vi "Node - Writer.vi"(8 "error in (no error)":errorcluster, 11 "Node Data In":T1) -> (0 "error out":errorcluster, 3 "Node Data Out":T1)   [LabVIEW 2016, in "PXImc Router.lvlib"]
uses:
  PXImc Router.lvlib
  Controls/Node Data.ctl
  Controls/Node/Node - PXImc Parameters.ctl
  Controls/Node/Node - Writer Data.ctl
  Controls/Node/Node Ch Properties.ctl
  Controls/Data Type.ctl
  Controls/Node/Node - Readers Data.ctl
  Controls/Node/Node - Reader Data.ctl
  Engine/PXImc Custom Device Engine.lvlib
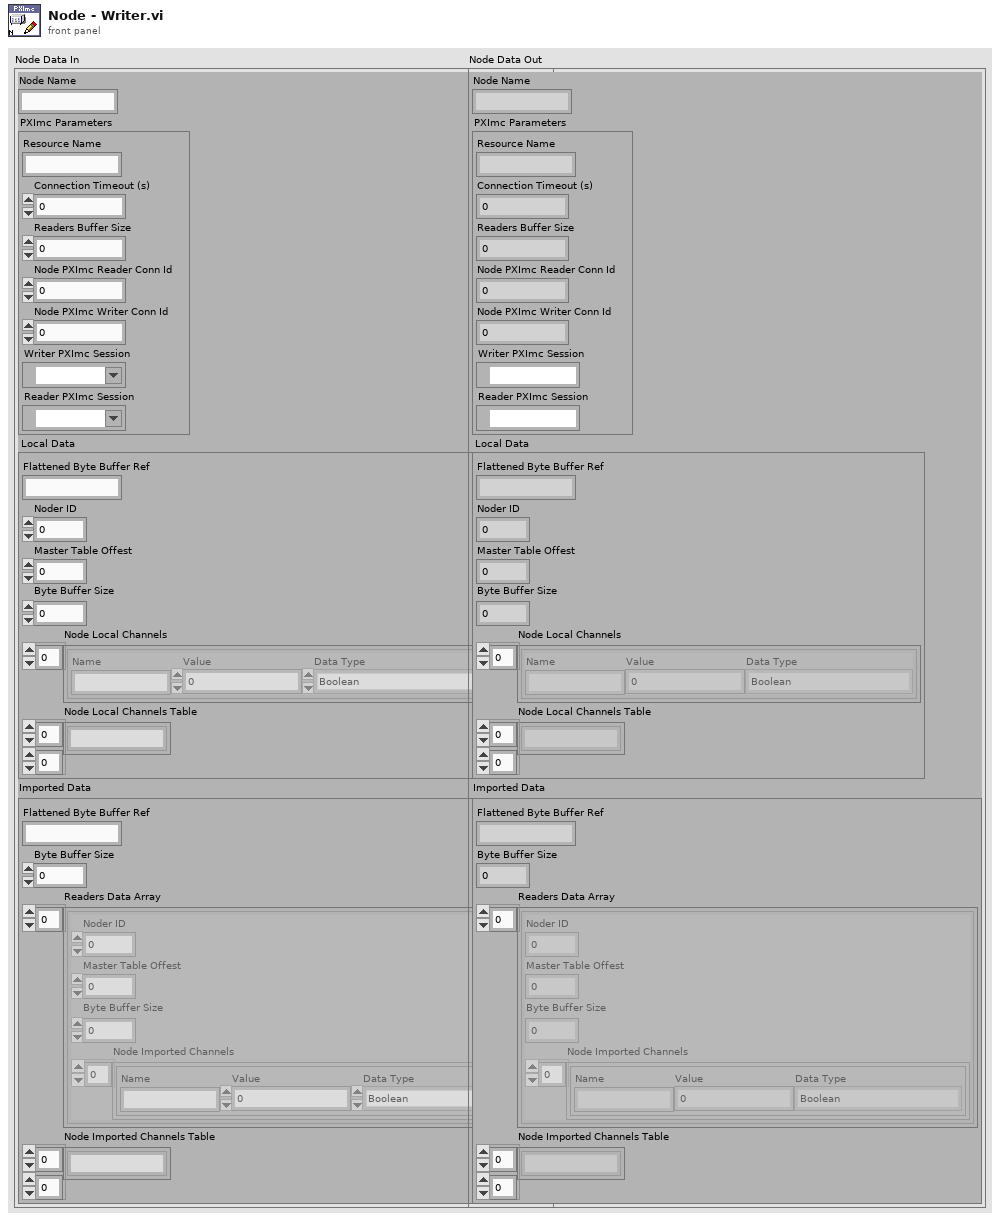
[diagram p1: front panel]
types:
  T1 = typedef "PXImc Router.lvlib/Node Data.ctl" = cluster{"Node Name":string, "PXImc Parameters":T2, "Local Data":T3, "Imported Data":T6}
  T2 = typedef "PXImc Router.lvlib/Node - PXImc Parameters.ctl" = cluster{"Resource Name":string, "Connection Timeout (s)":dbl, "Readers Buffer Size":u64, "Node PXImc Reader Conn Id":u16, "Node PXImc Writer Conn Id":u16, "Writer PXImc Session":refnum<k21>, "Reader PXImc Session":refnum<k21>}
  T3 = typedef "PXImc Router.lvlib/Node - Writer Data.ctl" = cluster{"Flattened Byte Buffer Ref":string, "Noder ID":u32, "Master Table Offest":u32, "Byte Buffer Size":u32, "Node Local Channels":T4[], "Node Local Channels Table":string[][]}
  T4 = typedef "PXImc Router.lvlib/Node Ch Properties.ctl" = cluster{"Name":string, "Value":dbl, "Data Type":T5}
  T5 = typedef "PXImc Router.lvlib/Data Type.ctl" = enum16{"Boolean", "SGL", "DBL", "I8", "I16", "I32", "I64", "U8", "U16", "U32", "U64"}
  T6 = typedef "PXImc Router.lvlib/Node - Readers Data.ctl" = cluster{"Flattened Byte Buffer Ref":string, "Byte Buffer Size":u64, "Readers Data Array":T7[], "Node Imported Channels Table":string[][]}
  T7 = typedef "PXImc Router.lvlib/Node - Reader Data.ctl" = cluster{"Noder ID":u32, "Master Table Offest":u32, "Byte Buffer Size":u64, "Node Imported Channels":T4[]}
  T8 = enum16{"Create File", "Log Message", "Log Error", "Log TimeStamp", "Close File"}
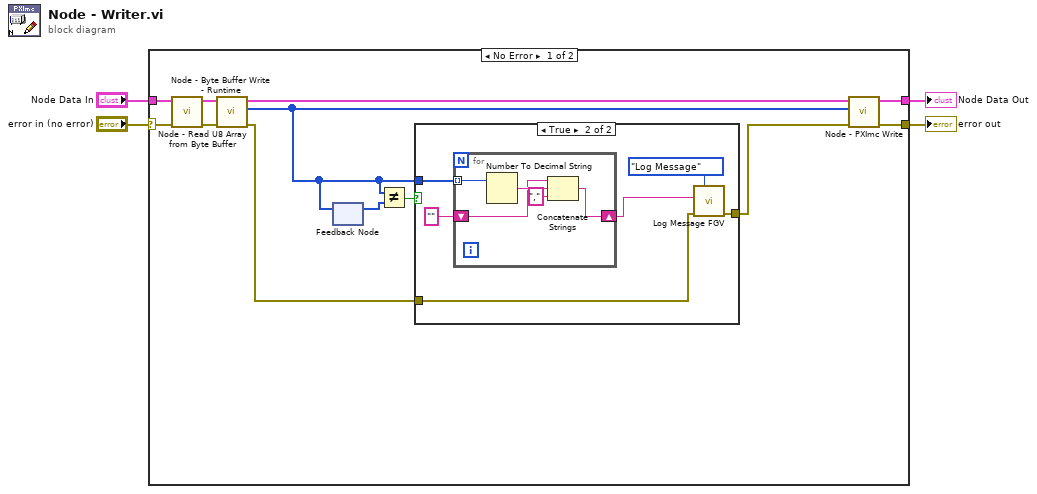
[diagram p0: block diagram]
diagram:
  n1 = case shown="No Error" "error in (no error)" {
    selector: "error in (no error)" -> [w12 w30]
    tunnel: [w16 w30] -> w4
    tunnel: "Node Data In" -> [w13 w29]
    tunnel: [w15 w29] -> w1
    frame No Error {
      n2 = call "Node - Byte Buffer Write - Runtime.vi"("error in (no error)"=w12, "Node Data In"=w13) -> ("error out"=w11:errorcluster, "Node Data Out"=w10:T1)  [unwired: 7 in, 1 out]
      n3 = call "Node - Read U8 Array from Byte Buffer.vi"("error in (no error)"=w11, "Node Data In"=w10) -> ("error out"=w7:errorcluster, "U8 Array Out"=w6:u8[], "Node Data Out"=w14:T1)  [unwired: 7 in]
      n4 = feedback #1() -> (w9:u8[])  [unwired: 1 in]
      n5 = feedback-in #1(w6) -> ()
      n6 = Not Equal?(x=w6, y=w9) -> (x != y?=w8:bool)
      n7 = case shown="True" w8 {
        tunnel: [w17 w22] -> w5
        tunnel: w6 -> [_ w19]
        tunnel: w7 -> [w17 w18]
        frame False {
        }
        frame True {
          n8 = for {
            shift-right: [w25] -> w20
            shift-left: "" -> [w24]
            tunnel: w19 -> [w28] mode=indexing
            n9 = Number To Decimal String(number=w28) -> (decimal integer string=w27:string)  [unwired: 1 in]
            n10 = Concatenate Strings(w24, w27, "," ("string")) -> (w25:string)
          }
          n11 = call "Log Message FGV.vi"("FGV Cmd"=T8."Log Message", "error in (no error)"=w18, "Message In"=w20) -> ("error out"=w22:errorcluster)  [unwired: 8 in]
        }
      }
      n12 = call "Node - PXImc Write.vi"("error in (no error)"=w5, "Writer Data In"=w6, "Node Data In"=w14) -> ("error out"=w16:errorcluster, "Node Data Out"=w15:T1)  [unwired: 7 in]
    }
    frame Error {
    }
  }
  "error out" <- w4
  "Node Data Out" <- w1
